vi "test_toml_reader.vi"(8 "error in (no error)":errorcluster, 11 "dragon_file_path":path=path "C:/Projects/toml-edit-labview/lv_src/test.toml") -> ()   [LabVIEW 2020]
uses:
  Item/type--enum.ctl
  Value/value_type--enum.ctl
  Doc/Doc.lvclass
  Table/Table.lvclass
  Item/Item.lvclass
  Value/Value.lvclass
  InlineTable/InlineTable.lvclass
panel:
  out "item_types":T1[](array[typedef])
  out "values":string[](array[string])
  out "value_types 2":T2[](array[typedef])
  out "item_names 2":string[](array[string])
  out "inline_table_item_names":string[](array[string])
  out "value_types":T2[](array[typedef])
  out "item_types":T1[](array[typedef])
  out "item_names":string[](array[string])
  out "value_strings":string[](array[string])
  out "item_names":string[](array[string])
  out "item_types":T1[](array[typedef])
  out "integer_value":i64
  out "string_value":string
  out "value_type":T2
  out "item_type":T1
  out "tables":string[](array[string])
  out "error out":errorcluster
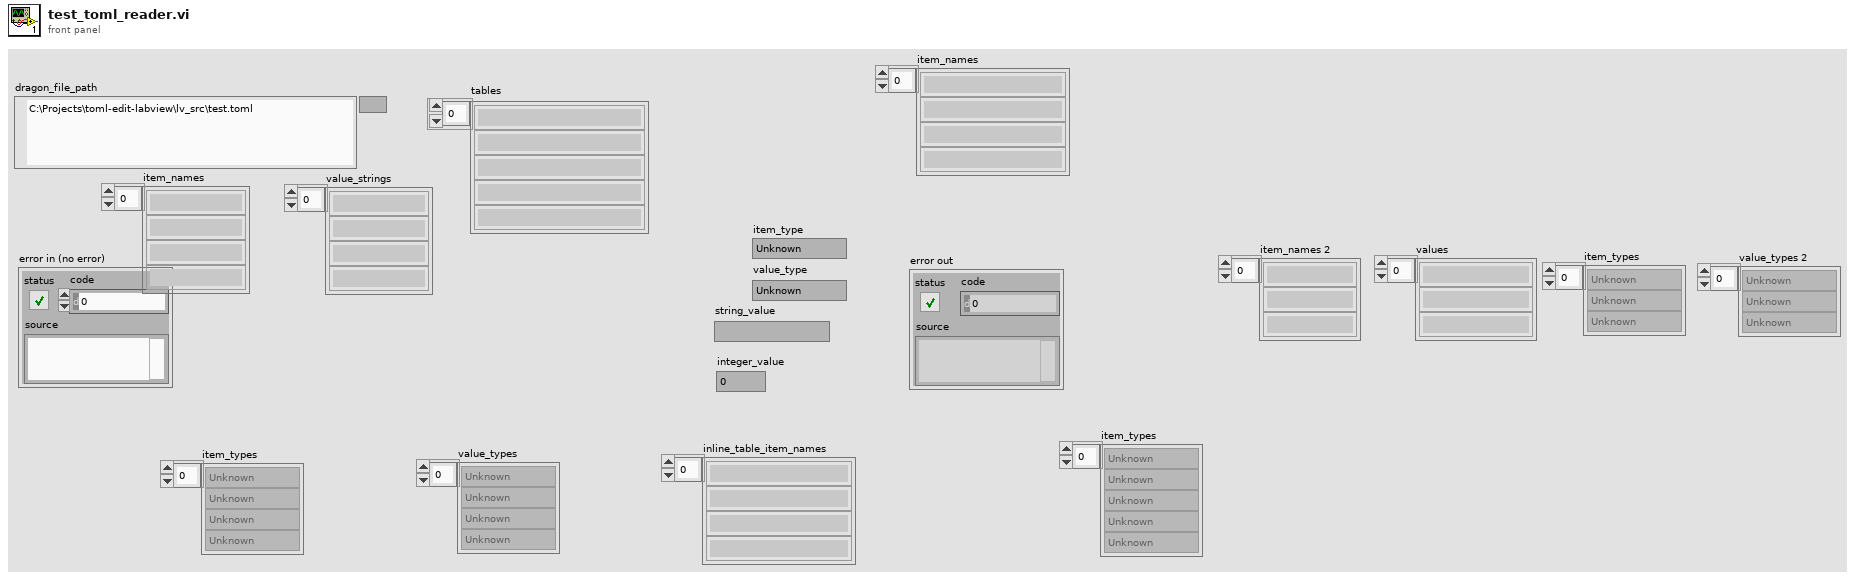
[diagram p1: front panel]
types:
  T1 = typedef "toml_edit.lvlib/Item.lvclass/type--enum.ctl" = enum16{"Unknown", "None", "Value", "ArrayOfTables", "Table"}
  T2 = typedef "toml_edit.lvlib/Value.lvclass/value_type--enum.ctl" = enum16{"Unknown", "String", "Integer", "Float", "Boolean", "Datetime", "Array", "InlineTable"}
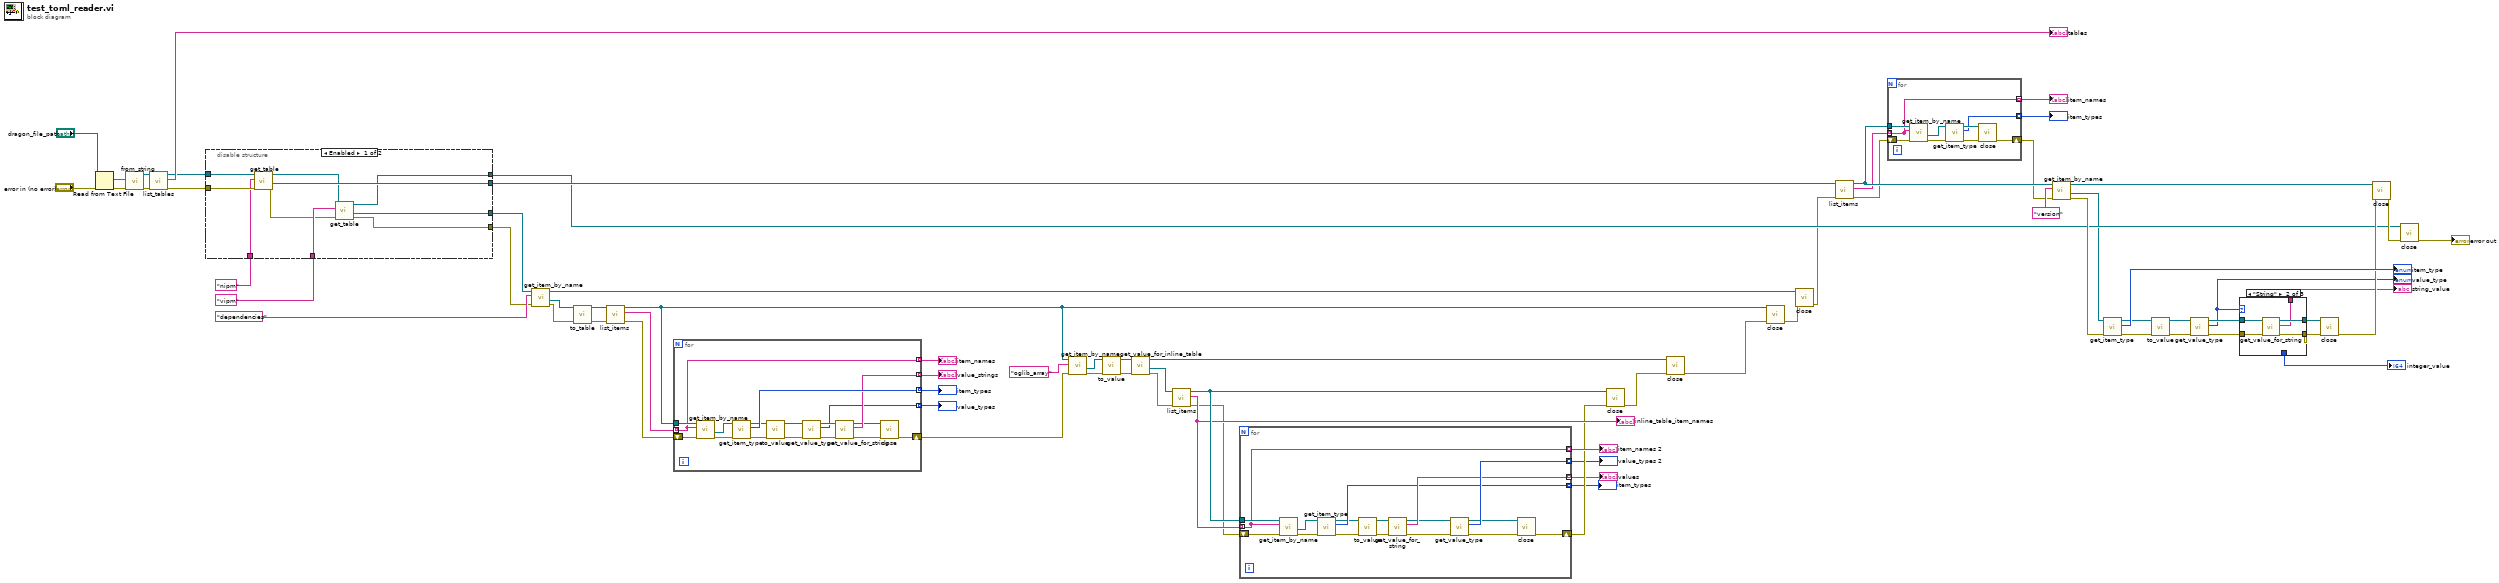
[diagram p0: block diagram]
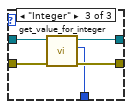
[diagram p3: hidden frame]
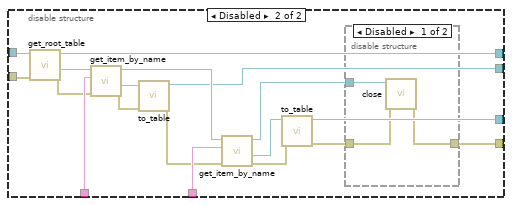
[diagram p4: hidden frame]
diagram:
  n1 = Read from Text File(file (use dialog)="dragon_file_path", error in="error in (no error)") -> (text=w71:string, error out=w70:errorcluster)  [unwired: 2 in, 2 out]
  n2 = call "from_string.vi"("error in (no error)"=w70, "toml"=w71) -> ("error out"=w68:errorcluster, "Doc out"=w69:refnum<class "Doc.lvclass">)  [unwired: 8 in]
  n3 = call "list_tables.vi"("error in (no error)"=w68, "Doc in"=w69) -> ("error out"=w65:errorcluster, "table_names"=→"tables":string[], "Doc out"=w66:refnum<class "Doc.lvclass">)  [unwired: 7 in]
  n4 = disable-structure shown="Enabled" {
    disable-tunnel: w66 -> [w84 w101]
    disable-tunnel: w65 -> [w83 w102]
    disable-tunnel: "nipm" ("table_name") -> [w82 w98]
    disable-tunnel: [w81 w94] -> w41
    disable-tunnel: [w79 w99] -> w40
    disable-tunnel: "vipm" ("table_name") -> [w78 w97]
    disable-tunnel: [w77 w92] -> w38
    disable-tunnel: [w76 w85] -> w20
    frame Enabled {
      n5 = call "get_table.vi"("error in (no error)"=w83, "table_name"=w82, "Doc in"=w84) -> ("error out"=w75:errorcluster, "Table"=w81:refnum<class "Table.lvclass">, "Doc out"=w80:refnum<class "Doc.lvclass">)  [unwired: 6 in]
      n6 = call "get_table.vi"("error in (no error)"=w75, "table_name"=w78, "Doc in"=w80) -> ("error out"=w76:errorcluster, "Table"=w77:refnum<class "Table.lvclass">, "Doc out"=w79:refnum<class "Doc.lvclass">)  [unwired: 6 in]
    }
    frame Disabled {
      n7 = call "get_root_table.vi"("error in (no error)"=w102, "Doc in"=w101) -> ("error out"=w88:errorcluster, "Table"=w100:refnum<class "Table.lvclass">, "Doc out"=w99:refnum<class "Doc.lvclass">)  [unwired: 7 in]
      n8 = call "get_item_by_name.vi"("error in (no error)"=w88, "item_name"=w98, "Table in"=w100) -> ("error out"=w89:errorcluster, "Item"=w95:refnum<class "Item.lvclass">, "Table out"=w96:refnum<class "Table.lvclass">)  [unwired: 6 in]
      n9 = call "to_table.vi"("error in (no error)"=w89, "Item in"=w95) -> ("error out"=w90:errorcluster, "Table"=w94:refnum<class "Table.lvclass">)  [unwired: 8 in]
      n10 = call "get_item_by_name.vi"("error in (no error)"=w90, "item_name"=w97, "Table in"=w96) -> ("error out"=w91:errorcluster, "Item"=w93:refnum<class "Item.lvclass">, "Table out"=w87:refnum<class "Table.lvclass">)  [unwired: 6 in]
      n11 = call "to_table.vi"("error in (no error)"=w91, "Item in"=w93) -> ("error out"=w86:errorcluster, "Table"=w92:refnum<class "Table.lvclass">)  [unwired: 8 in]
      n12 = disable-structure shown="Disabled" {
        disable-tunnel: w87 -> [w105 _]
        disable-tunnel: w86 -> [w104 w106]
        disable-tunnel: [w103 w106] -> w85
        frame Disabled {
          n13 = call "close.vi"("error in (no error)"=w104, "Table in"=w105) -> ("error out"=w103:errorcluster)  [unwired: 9 in]
        }
        frame Enabled {
        }
      }
    }
  }
  n14 = call "get_item_by_name.vi"("error in (no error)"=w20, "item_name"="dependencies" ("table_name"), "Table in"=w38) -> ("error out"=w35:errorcluster, "Item"=w19:refnum<class "Item.lvclass">, "Table out"=w33:refnum<class "Table.lvclass">)  [unwired: 6 in]
  n15 = call "to_table.vi"("error in (no error)"=w35, "Item in"=w19) -> ("error out"=w36:errorcluster, "Table"=w22:refnum<class "Table.lvclass">)  [unwired: 8 in]
  n16 = call "list_items.vi"("error in (no error)"=w36, "Table in"=w22) -> ("error out"=w30:errorcluster, "items"=w31:string[], "Table out"=w25:refnum<class "Table.lvclass">)  [unwired: 7 in]
  n17 = for {
    tunnel: w25 -> [w123]
    tunnel: w31 -> [w119] mode=indexing
    shift-right: [w113] -> w24
    shift-left: w30 -> [w122]
    tunnel: [w120] -> w27 mode=indexing
    tunnel: [w119] -> w28 mode=indexing
    tunnel: [w116] -> w29 mode=indexing
    tunnel: [w109] -> w26 mode=indexing
    n18 = call "get_item_by_name.vi"("error in (no error)"=w122, "item_name"=w119, "Table in"=w123) -> ("error out"=w121:errorcluster, "Item"=w107:refnum<class "Item.lvclass">)  [unwired: 6 in, 1 out]
    n19 = call "get_item_type.vi"("error in (no error)"=w121, "Item in"=w107) -> ("error out"=w117:errorcluster, "item_type"=w120:T1, "Item out"=w118:refnum<class "Item.lvclass">)  [unwired: 7 in]
    n20 = call "to_value.vi"("error in (no error)"=w117, "Item in"=w118) -> ("error out"=w111:errorcluster, "Value out"=w108:refnum<class "Value.lvclass">)  [unwired: 8 in]
    n21 = call "get_value_type.vi"("error in (no error)"=w111, "Value in"=w108) -> ("error out"=w110:errorcluster, "value_type"=w109:T2, "Value out"=w112:refnum<class "Value.lvclass">)  [unwired: 6 in, 1 out]
    n22 = call "get_value_for_string.vi"("error in (no error)"=w110, "Value in"=w112) -> ("error out"=w115:errorcluster, "string_value"=w116:string, "Value out"=w114:refnum<class "Value.lvclass">)  [unwired: 7 in]
    n23 = call "close.vi"("error in (no error)"=w115, "Value in"=w114) -> ("error out"=w113:errorcluster)  [unwired: 9 in]
  }
  "value_strings" <- w29
  "item_names" <- w28
  "item_types" <- w27
  "value_types" <- w26
  n24 = call "get_item_by_name.vi"("error in (no error)"=w24, "item_name"="oglib_array", "Table in"=w25) -> ("error out"=w16:errorcluster, "Item"=w2:refnum<class "Item.lvclass">)  [unwired: 6 in, 1 out]
  n25 = call "to_value.vi"("error in (no error)"=w16, "Item in"=w2) -> ("error out"=w15:errorcluster, "Value out"=w13:refnum<class "Value.lvclass">)  [unwired: 8 in]
  n26 = call "get_value_for_inline_table.vi"("error in (no error)"=w15, "Value in"=w13) -> ("error out"=w12:errorcluster, "InlineTable out"=w1:refnum<class "InlineTable.lvclass">, "Value out"=w14:refnum<class "Value.lvclass">)  [unwired: 7 in]
  n27 = call "list_items.vi"("error in (no error)"=w12, "Table in"=w1) -> ("error out"=w7:errorcluster, "items"=w8:string[], "Table out"=w9:refnum<class "InlineTable.lvclass">)  [unwired: 7 in]
  "inline_table_item_names" <- w8
  n28 = for {
    tunnel: w9 -> [w140]
    tunnel: w8 -> [w137] mode=indexing
    shift-right: [w138] -> w6
    shift-left: w7 -> [w139]
    tunnel: [w137] -> w10 mode=indexing
    tunnel: [w136] -> w5 mode=indexing
    tunnel: [w135] -> w4 mode=indexing
    tunnel: [w134] -> w3 mode=indexing
    n29 = call "get_item_by_name.vi"("error in (no error)"=w139, "key_name"=w137, "Table in"=w140) -> ("error out"=w129:errorcluster, "Item"=w124:refnum<class "Item.lvclass">)  [unwired: 6 in, 1 out]
    n30 = call "get_item_type.vi"("error in (no error)"=w129, "Item in"=w124) -> ("error out"=w128:errorcluster, "item_type"=w134:T1, "Item out"=w126:refnum<class "Item.lvclass">)  [unwired: 7 in]
    n31 = call "to_value.vi"("error in (no error)"=w128, "Item in"=w126) -> ("error out"=w127:errorcluster, "Value out"=w125:refnum<class "Value.lvclass">)  [unwired: 8 in]
    n32 = call "get_value_for_string.vi"("error in (no error)"=w127, "Value in"=w125) -> ("error out"=w131:errorcluster, "string_value"=w135:string, "Value out"=w130:refnum<class "Value.lvclass">)  [unwired: 7 in]
    n33 = call "get_value_type.vi"("error in (no error)"=w131, "Value in"=w130) -> ("error out"=w133:errorcluster, "value_type"=w136:T2, "Value out"=w132:refnum<class "Value.lvclass">)  [unwired: 6 in, 1 out]
    n34 = call "close.vi"("error in (no error)"=w133, "Value in"=w132) -> ("error out"=w138:errorcluster)  [unwired: 9 in]
  }
  "item_names 2" <- w10
  "value_types 2" <- w5
  "values" <- w4
  "item_types" <- w3
  n35 = call "close.vi"("error in (no error)"=w6, "Table in"=w9) -> ("error out"=w11:errorcluster)  [unwired: 9 in]
  n36 = call "close.vi"("error in (no error)"=w11, "Value in"=w14) -> ("error out"=w23:errorcluster)  [unwired: 9 in]
  n37 = call "close.vi"("error in (no error)"=w23, "Table in"=w25) -> ("error out"=w34:errorcluster)  [unwired: 9 in]
  n38 = call "close.vi"("error in (no error)"=w34, "Table in"=w33) -> ("error out"=w32:errorcluster)  [unwired: 9 in]
  n39 = call "list_items.vi"("error in (no error)"=w32, "Table in"=w41) -> ("error out"=w44:errorcluster, "items"=w46:string[], "Table out"=w47:refnum<class "Table.lvclass">)  [unwired: 7 in]
  n40 = for {
    tunnel: w47 -> [w149]
    tunnel: w46 -> [w142] mode=indexing
    shift-right: [w144] -> w43
    shift-left: w44 -> [w148]
    tunnel: [w143] -> w45 mode=indexing
    tunnel: [w142] -> w42 mode=indexing
    n41 = call "get_item_by_name.vi"("error in (no error)"=w148, "item_name"=w142, "Table in"=w149) -> ("error out"=w147:errorcluster, "Item"=w141:refnum<class "Item.lvclass">)  [unwired: 6 in, 1 out]
    n42 = call "get_item_type.vi"("error in (no error)"=w147, "Item in"=w141) -> ("error out"=w145:errorcluster, "item_type"=w143:T1, "Item out"=w146:refnum<class "Item.lvclass">)  [unwired: 7 in]
    n43 = call "close.vi"("error in (no error)"=w145, "Item in"=w146) -> ("error out"=w144:errorcluster)  [unwired: 9 in]
  }
  "item_types" <- w45
  "item_names" <- w42
  n44 = call "get_item_by_name.vi"("error in (no error)"=w43, "item_name"="version", "Table in"=w47) -> ("error out"=w62:errorcluster, "Item"=w18:refnum<class "Item.lvclass">, "Table out"=w60:refnum<class "Table.lvclass">)  [unwired: 6 in]
  n45 = call "get_item_type.vi"("error in (no error)"=w62, "Item in"=w18) -> ("error out"=w57:errorcluster, "item_type"=→"item_type":T1, "Item out"=w58:refnum<class "Item.lvclass">)  [unwired: 7 in]
  n46 = call "to_value.vi"("error in (no error)"=w57, "Item in"=w58) -> ("error out"=w56:errorcluster, "Value out"=w21:refnum<class "Value.lvclass">)  [unwired: 8 in]
  n47 = call "get_value_type.vi"("error in (no error)"=w56, "Value in"=w21) -> ("error out"=w53:errorcluster, "value_type"=w49:T2, "Value out"=w54:refnum<class "Value.lvclass">)  [unwired: 6 in, 1 out]
  "value_type" <- w49
  n48 = case shown="\"String\"" w49 {
    tunnel: w54 -> [w151 w156 w161]
    tunnel: w53 -> [w150 w155 w160]
    tunnel: [w150 w154 w159] -> w52
    tunnel: [w151 w153 w158] -> w51
    tunnel: [_ w152 _] -> w50
    tunnel: [_ _ w157] -> w48
    frame Default {
    }
    frame "String" {
      n49 = call "get_value_for_string.vi"("error in (no error)"=w155, "Value in"=w156) -> ("error out"=w154:errorcluster, "string_value"=w152:string, "Value out"=w153:refnum<class "Value.lvclass">)  [unwired: 7 in]
    }
    frame "Integer" {
      n50 = call "get_value_for_integer.vi"("error in (no error)"=w160, "Value in"=w161) -> ("error out"=w159:errorcluster, "integer_value"=w157:i64, "Value out"=w158:refnum<class "Value.lvclass">)  [unwired: 7 in]
    }
  }
  "string_value" <- w50
  "integer_value" <- w48
  n51 = call "close.vi"("error in (no error)"=w52, "Value in"=w51) -> ("error out"=w55:errorcluster)  [unwired: 9 in]
  n52 = call "close.vi"("error in (no error)"=w55, "Table in"=w60) -> ("error out"=w63:errorcluster)  [unwired: 9 in]
  n53 = call "close.vi"("error in (no error)"=w63, "Doc in"=w40) -> ("error out"=→"error out":errorcluster)  [unwired: 9 in]
